vi "Preset subsystems.vi"(10 "appended array":bool[](array[boolean]), 11 "Enum":T1(ring)=enum."Low Hatch") -> ()   [LabVIEW 2018]
uses:
  5daef287-ccd4-4bc1-8e60-40fa11514e16.vi
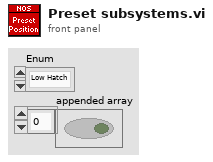
[diagram p1: front panel]
types:
  T1 = enum16{"Pick Up Ball", "Pick Up Hatch", "Shoot Ball", "Shoot Hatch", "Low Ball", "Middle Ball", "High Ball", "High Hatch", "Middle Hatch", "Low Hatch", "Cargo Ball", "Ball Loading Station", "Ball Ground", "Reserve"}
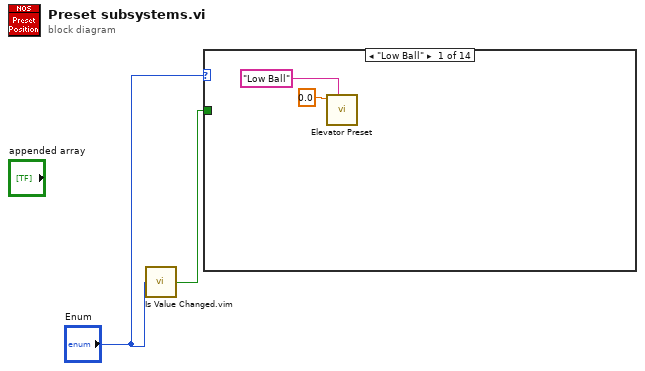
[diagram p0: block diagram]
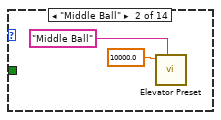
[diagram p2: hidden frame]
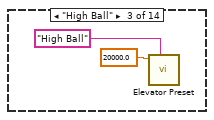
[diagram p3: hidden frame]
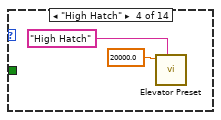
[diagram p4: hidden frame]
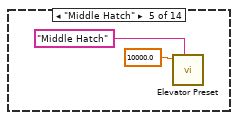
[diagram p5: hidden frame]
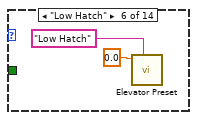
[diagram p6: hidden frame]
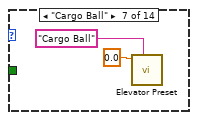
[diagram p7: hidden frame]
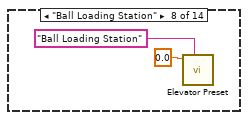
[diagram p8: hidden frame]
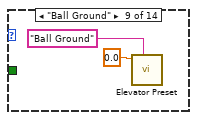
[diagram p9: hidden frame]
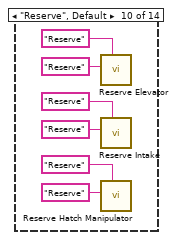
[diagram p10: hidden frame]
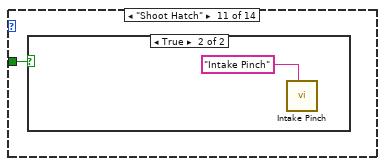
[diagram p11: hidden frame]
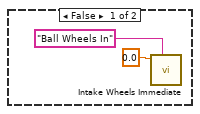
[diagram p12: hidden frame]
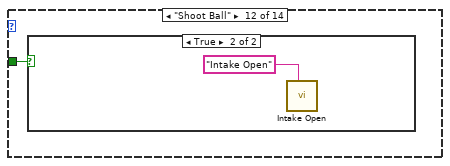
[diagram p13: hidden frame]
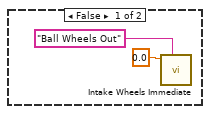
[diagram p14: hidden frame]
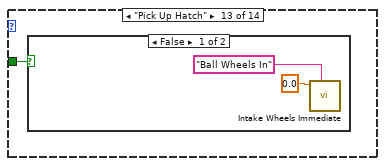
[diagram p15: hidden frame]
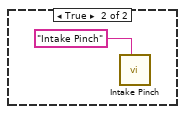
[diagram p16: hidden frame]
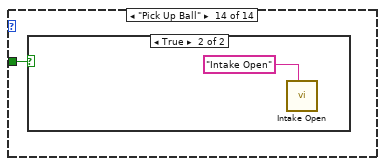
[diagram p17: hidden frame]
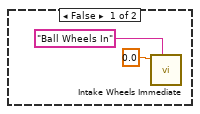
[diagram p18: hidden frame]
diagram:
  n1 = call "Is Value Changed.vim"("value"="Enum") -> ("changed or first call?"=w1:bool)
  n2 = case shown="\"Low Ball\"" "Enum" {
    tunnel: w1 -> [_ _ _ _ _ _ _ _ _ _ w27 w31 w35 w39]
    frame "Low Ball" {
      n3 = call "Elevator Preset.vi"("Description"="Low Ball", "Position"=0.0) -> ()  [unwired: 9 in, 1 out]
    }
    frame "Middle Ball" {
      n4 = call "Elevator Preset.vi"("Description"="Middle Ball", "Position"=10000.0) -> ()  [unwired: 9 in, 1 out]
    }
    frame "High Ball" {
      n5 = call "Elevator Preset.vi"("Description"="High Ball", "Position"=20000.0) -> ()  [unwired: 9 in, 1 out]
    }
    frame "High Hatch" {
      n6 = call "Elevator Preset.vi"("Description"="High Hatch", "Position"=20000.0) -> ()  [unwired: 9 in, 1 out]
    }
    frame "Middle Hatch" {
      n7 = call "Elevator Preset.vi"("Description"="Middle Hatch", "Position"=10000.0) -> ()  [unwired: 9 in, 1 out]
    }
    frame "Low Hatch" {
      n8 = call "Elevator Preset.vi"("Description"="Low Hatch", "Position"=0.0) -> ()  [unwired: 9 in, 1 out]
    }
    frame "Cargo Ball" {
      n9 = call "Elevator Preset.vi"("Description"="Cargo Ball", "Position"=0.0) -> ()  [unwired: 9 in, 1 out]
    }
    frame "Ball Loading Station" {
      n10 = call "Elevator Preset.vi"("Description"="Ball Loading Station", "Position"=0.0) -> ()  [unwired: 9 in, 1 out]
    }
    frame "Ball Ground" {
      n11 = call "Elevator Preset.vi"("Description"="Ball Ground", "Position"=0.0) -> ()  [unwired: 9 in, 1 out]
    }
    frame "Reserve", Default {
      n12 = call "Reserve Elevator.vi"("Description"="Reserve", "Command Name"="Reserve") -> ()  [unwired: 9 in, 1 out]
      n13 = call "Reserve Intake.vi"("Description"="Reserve", "Command Name"="Reserve") -> ()  [unwired: 9 in, 1 out]
      n14 = call "Reserve Hatch Manipulator.vi"("Description"="Reserve", "Command Name"="Reserve") -> ()  [unwired: 9 in, 1 out]
    }
    frame "Shoot Hatch" {
      n15 = case shown="True" w27 {
        frame False {
          n16 = call "Intake Wheels Immediate.vi"("Description"="Ball Wheels In", "Setpoint"=0.0) -> ()  [unwired: 9 in, 1 out]
        }
        frame True {
          n17 = call "Intake Pinch.vi"("Description"="Intake Pinch") -> ()  [unwired: 10 in, 1 out]
        }
      }
    }
    frame "Shoot Ball" {
      n18 = case shown="True" w31 {
        frame False {
          n19 = call "Intake Wheels Immediate.vi"("Description"="Ball Wheels Out", "Setpoint"=0.0) -> ()  [unwired: 9 in, 1 out]
        }
        frame True {
          n20 = call "Intake Open.vi"("Description"="Intake Open") -> ()  [unwired: 10 in, 1 out]
        }
      }
    }
    frame "Pick Up Hatch" {
      n21 = case shown="False" w35 {
        frame False {
          n22 = call "Intake Wheels Immediate.vi"("Description"="Ball Wheels In", "Setpoint"=0.0) -> ()  [unwired: 9 in, 1 out]
        }
        frame True {
          n23 = call "Intake Pinch.vi"("Description"="Intake Pinch") -> ()  [unwired: 10 in, 1 out]
        }
      }
    }
    frame "Pick Up Ball" {
      n24 = case shown="True" w39 {
        frame False {
          n25 = call "Intake Wheels Immediate.vi"("Description"="Ball Wheels In", "Setpoint"=0.0) -> ()  [unwired: 9 in, 1 out]
        }
        frame True {
          n26 = call "Intake Open.vi"("Description"="Intake Open") -> ()  [unwired: 10 in, 1 out]
        }
      }
    }
  }
